vi "Add Offline Data Folder.vi"(8 "error in (no error)":errorcluster, 11 "Node Ptr":T1=18446744073709551615 format="%.0x") -> (0 "error out":errorcluster)   [LabVIEW 2017, in "OPC UA Client System Explorer.lvlib"]
uses:
  OPC UA Client System Explorer.lvlib
  <vilib>/NI Veristand/Custom Device API/Custom Device Item Ref.ctl
  Shared/Constants.vi
  Shared/OPC UA Client Shared.lvlib
  <vilib>/NI VeriStand/Custom Device API/Custom Device API.lvlib
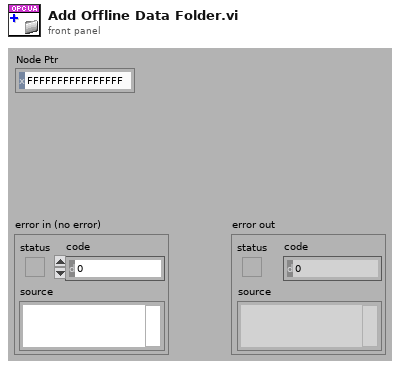
[diagram p1: front panel]
types:
  T1 = typedef "Custom Device API.lvlib/Custom Device Item Ref.ctl" = u64
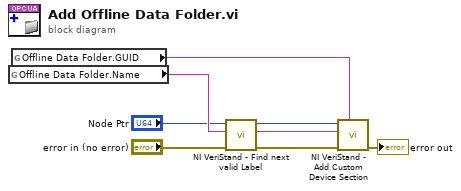
[diagram p0: block diagram]
diagram:
  n1 = global read "Constants.vi" "Offline Data Folder.Name"() -> (w6:string)
  n2 = global read "Constants.vi" "Offline Data Folder.GUID"() -> (w7:string)
  n3 = call <vilib>:"NI VeriStand - Find next valid Label.vi"("error in (no error)"="error in (no error)", "Label"=w6, "Item Ref in"="Node Ptr") -> ("error out"=w2:errorcluster, "Label out"=w1:string, "Item Ref out"=w4:T1)  [unwired: 4 in, 2 out]
  n4 = call <vilib>:"NI VeriStand - Add Custom Device Section.vi"("GUID (Default Section)"=w7, "error in (no error)"=w2, "Section Name"=w1, "Parent Ref in"=w4) -> ("error out"=→"error out":errorcluster)  [unwired: 4 in, 3 out]
